vi "UpdateVandAGlobals.vi"(3 "ByPass Pop up?":bool, 4 "Motion Settings":T1={"No Motion?"=FALSE, "Motion System"=enum."NI 735x", "Motion Bd ID"=1, "Motion Profile"="SMAC1", "# Axis"=1, "Reverse Z axis?"=TRUE, "SMAC Axis"=0, "scan pair"=enum."y-(x) scan", "RT fps"=6.0, "Steps per mm"=[1000, 1000, 1000, 1000], "Motor Parameters"={"velocity ct/s"=[10000.0, 10000.0, 10000.0, 50000.0], "accel ct/s^2"=[50000.0, 50000.0, 50000.0, 200000.0]}, "One Way Scan"=FALSE, "Reverse One Way Scan"=FALSE, "Global Position (mm)"=[], "Plane"=0, "Distance between\nscan lines (um)"=0.0, "Distance between\nscan planes (um)"=0.0, "number of scan planes"=1, "Total steps in line"=0, "Xtra plane\ndistance  (um)"=100, "Xtra planes "=1, "Add Axis"=FALSE, "overshoot cts"=200, "BKPT Shift"=0, "Scan Start Time (ms)"=0, "ESP VISA"="GPIB::1::INSTR", "3rd Axis"=1, "GL Ref Out"=refnum, "Galil Address"=""} {"3rd Axis" items=["x", "y", "z", "w"]; "Xtra planes" min=1; "Xtra plane\ndistance  (um)" min=0; "Distance between\nscan planes (um)" format="%.2f"; "Distance between\nscan lines (um)" format="%.2f"; "SMAC Axis" items=["None"=0, "Axis 1"=1, "Axis 2"=2, "Axis 3"=3, "Axis 4"=4, "Axis 5"=5, "Axis 6"=6, "Axis 7"=7, "Axis 8"=8, "Vector Space 1"=17, "Vector Space 2"=18, "Vector Space 3"=19, "Vector Space 4"=20]; "Motion Bd ID" min=1 max=32 step=1}) -> (1 "Motion Settings Out":T1={"No Motion?"=FALSE, "Motion System"=enum."NI 735x", "Motion Bd ID"=1, "Motion Profile"="SMAC1", "# Axis"=1, "Reverse Z axis?"=TRUE, "SMAC Axis"=0, "scan pair"=enum."y-(x) scan", "RT fps"=6.0, "Steps per mm"=[1000, 1000, 1000, 1000], "Motor Parameters"={"velocity ct/s"=[10000.0, 10000.0, 10000.0, 50000.0], "accel ct/s^2"=[50000.0, 50000.0, 50000.0, 200000.0]}, "One Way Scan"=FALSE, "Reverse One Way Scan"=FALSE, "Global Position (mm)"=[], "Plane"=0, "Distance between\nscan lines (um)"=0.0, "Distance between\nscan planes (um)"=0.0, "number of scan planes"=1, "Total steps in line"=0, "Xtra plane\ndistance  (um)"=100, "Xtra planes "=1, "Add Axis"=FALSE, "overshoot cts"=200, "BKPT Shift"=0, "Scan Start Time (ms)"=0, "ESP VISA"="GPIB::1::INSTR", "3rd Axis"=1, "GL Ref Out"=refnum, "Galil Address"=""} {"3rd Axis" items=["x", "y", "z", "w"]; "Xtra planes" min=1; "Xtra plane\ndistance  (um)" min=0; "Distance between\nscan planes (um)" format="%.2f"; "Distance between\nscan lines (um)" format="%.2f"; "SMAC Axis" items=["None"=0, "Axis 1"=1, "Axis 2"=2, "Axis 3"=3, "Axis 4"=4, "Axis 5"=5, "Axis 6"=6, "Axis 7"=7, "Axis 8"=8, "Vector Space 1"=17, "Vector Space 2"=18, "Vector Space 3"=19, "Vector Space 4"=20]; "Motion Bd ID" min=1 max=32 step=1}, 2 "Motor Parameters":T5)   [LabVIEW 2022 SP3]
uses:
  MotionParameters.ctl
  MotionSys.ctl
  -MotionRoutines/ScanAxis.ctl
  -MotionRoutines/3rdAxis.ctl
panel:
  in  "stop":bool
  in  "Select Motor Parameters":T6
  # "1-D and 2-D B scan settings"
  # "1-D and 2-D B scan settings"
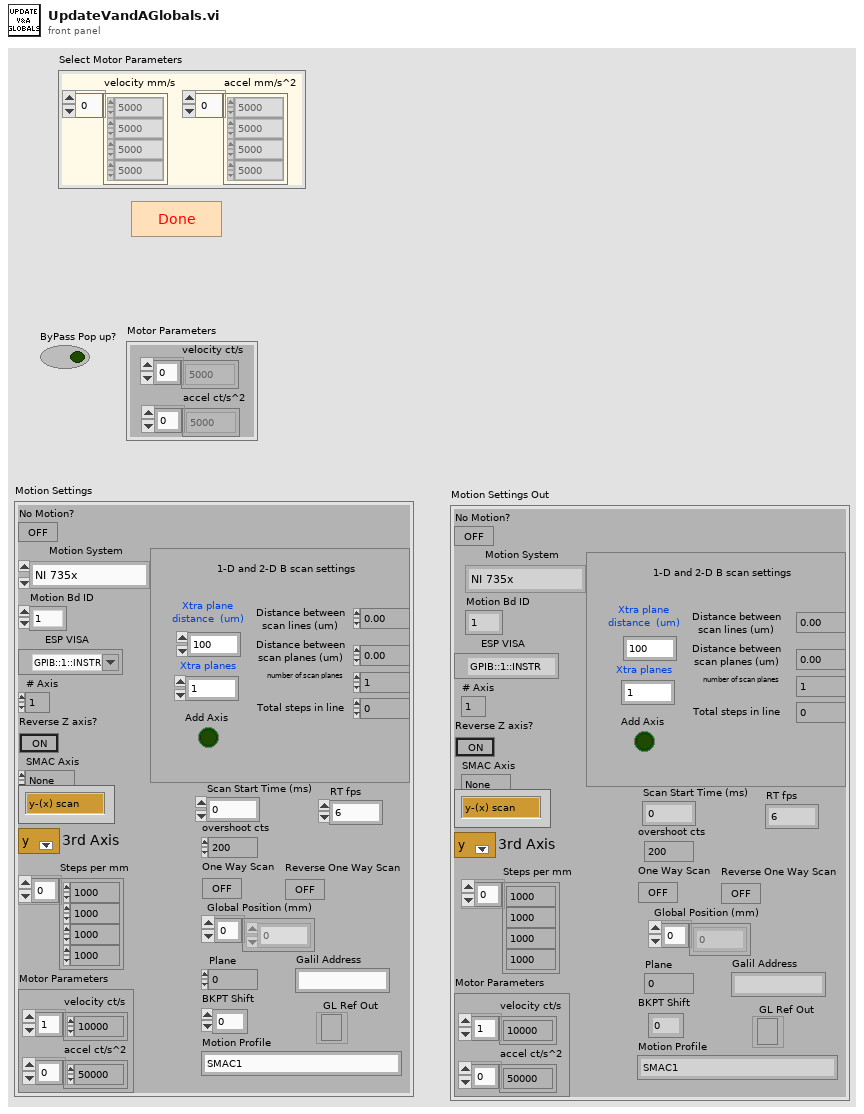
[diagram p1: front panel]
types:
  T1 = typedef "MotionParameters.ctl" = cluster{"No Motion?":bool, "Motion System":T2, "Motion Bd ID":u8, "Motion Profile":string, "# Axis":i8, "Reverse Z axis?":bool, "SMAC Axis":u16, "scan pair":T3, "RT fps":sgl, "Steps per mm":i32[], "Motor Parameters":cluster{"velocity ct/s":dbl[], "accel ct/s^2":dbl[]}, "One Way Scan":bool, "Reverse One Way Scan":bool, "Global Position (mm)":dbl[], "Plane":i32, "Distance between\nscan lines (um)":sgl, "Distance between\nscan planes (um)":sgl, "number of scan planes":i32, "Total steps in line":i32, "Xtra plane\ndistance  (um)":i32, "Xtra planes ":i32, "Add Axis":bool, "overshoot cts":i32, "BKPT Shift":i32, "Scan Start Time (ms)":u32, "ESP VISA":refnum<visa-resource-name>, "3rd Axis":T4, "GL Ref Out":refnum<k7>, "Galil Address":string}
  T2 = typedef "MotionSys.ctl" = enum16{"MM3000", "NI 735x", "Newport ESP", "No Motion Card", "Galil"}
  T3 = typedef "ScanAxis.ctl" = enum16{"y-(x) scan", "x-(y) scan", "z-(x) scan", "z-(y) scan", "y-(z) scan", "x-(z) scan", "w-(x) scan", "w-(y) scan", "w-(z) scan", "x-(w) scan", "y-(w) scan", "z-(w) scan"}
  T4 = typedef "3rdAxis.ctl" = u16
  T5 = cluster{"velocity ct/s":i32[], "accel ct/s^2":i32[]}
  T6 = cluster{"velocity mm/s":dbl[], "accel mm/s^2":dbl[]}
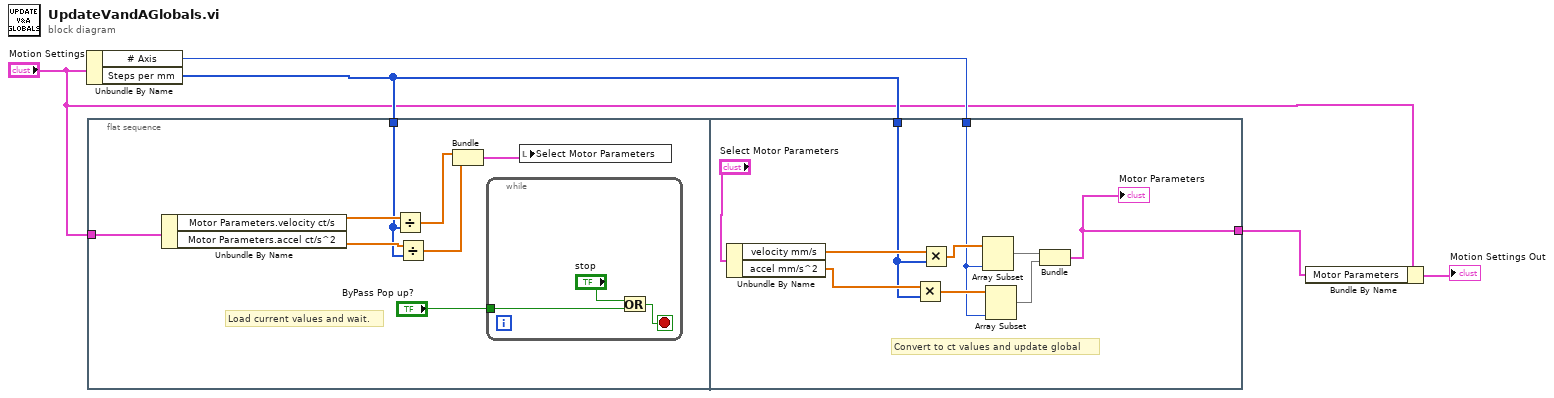
[diagram p0: block diagram]
diagram:
  n1 = Unbundle By Name("Motion Settings") -> ("# Axis"=w4:i8, "Steps per mm"=w5:i32[])
  n2 = flat-sequence {
    tunnel: w5 -> [w11]
    tunnel: "Motion Settings" -> [w7]
    tunnel: w5 -> [w19]
    tunnel: w4 -> [w18]
    tunnel: [w17] -> w2
    frame #0 {
      # "Load current values and wait."
      n3 = Unbundle By Name(w7) -> ("Motor Parameters.velocity ct/s"=w13:dbl[], "Motor Parameters.accel ct/s^2"=w12:dbl[])
      n4 = Divide(x=w13, y=w11) -> (x/y=w10:dbl[])
      n5 = Divide(x=w12, y=w11) -> (x/y=w9:dbl[])
      n6 = Bundle(w10, w9) -> (w8:cluster{dbl[], dbl[]})  [unwired: 1 in]
      n7 = while {
        tunnel: "ByPass Pop up?" -> [w14]
        stop <- w16 stop-if-true
        n8 = Or(x="stop", y=w14) -> (x .or. y?=w16:bool)
      }
      n9 = local write "Select Motor Parameters"(w8) -> ()
    }
    frame #1 {
      # "Convert to ct values and update global"
      n10 = Unbundle By Name("Select Motor Parameters") -> ("velocity mm/s"=w26:dbl[], "accel mm/s^2"=w25:dbl[])
      n11 = Multiply(x=w25, y=w19) -> (x*y=w23:dbl[])
      n12 = Multiply(x=w26, y=w19) -> (x*y=w24:dbl[])
      n13 = Array Subset(array=w24, length=w18) -> (w22:dbl[])  [unwired: 1 in]
      n14 = Array Subset(array=w23, length=w18) -> (w21:dbl[])  [unwired: 1 in]
      n15 = Bundle(w22, w21) -> (w17:cluster{dbl[], dbl[]})  [unwired: 1 in]
      "Motor Parameters" <- w17
    }
  }
  n16 = Bundle By Name(cluster="Motion Settings", "Motor Parameters"=w2) -> (→"Motion Settings Out":T1)
